vi "ImportScan.vi"(8 "error in (no error)":errorcluster, 9 "reference":refnum<vi>, 11 "Database in":refnum<class "Database.lvclass">) -> (0 "error out":errorcluster, 1 "reference 2":refnum<vi>, 3 "Database out":refnum<class "Database.lvclass">)   [LabVIEW 2014, in "Database.lvclass"]
uses:
  Database.lvclass
  Database.lvclass/Database.ctl
  <vilib>/addons/database/NI_Database_API.lvlib
panel:
  in  "scan":T1
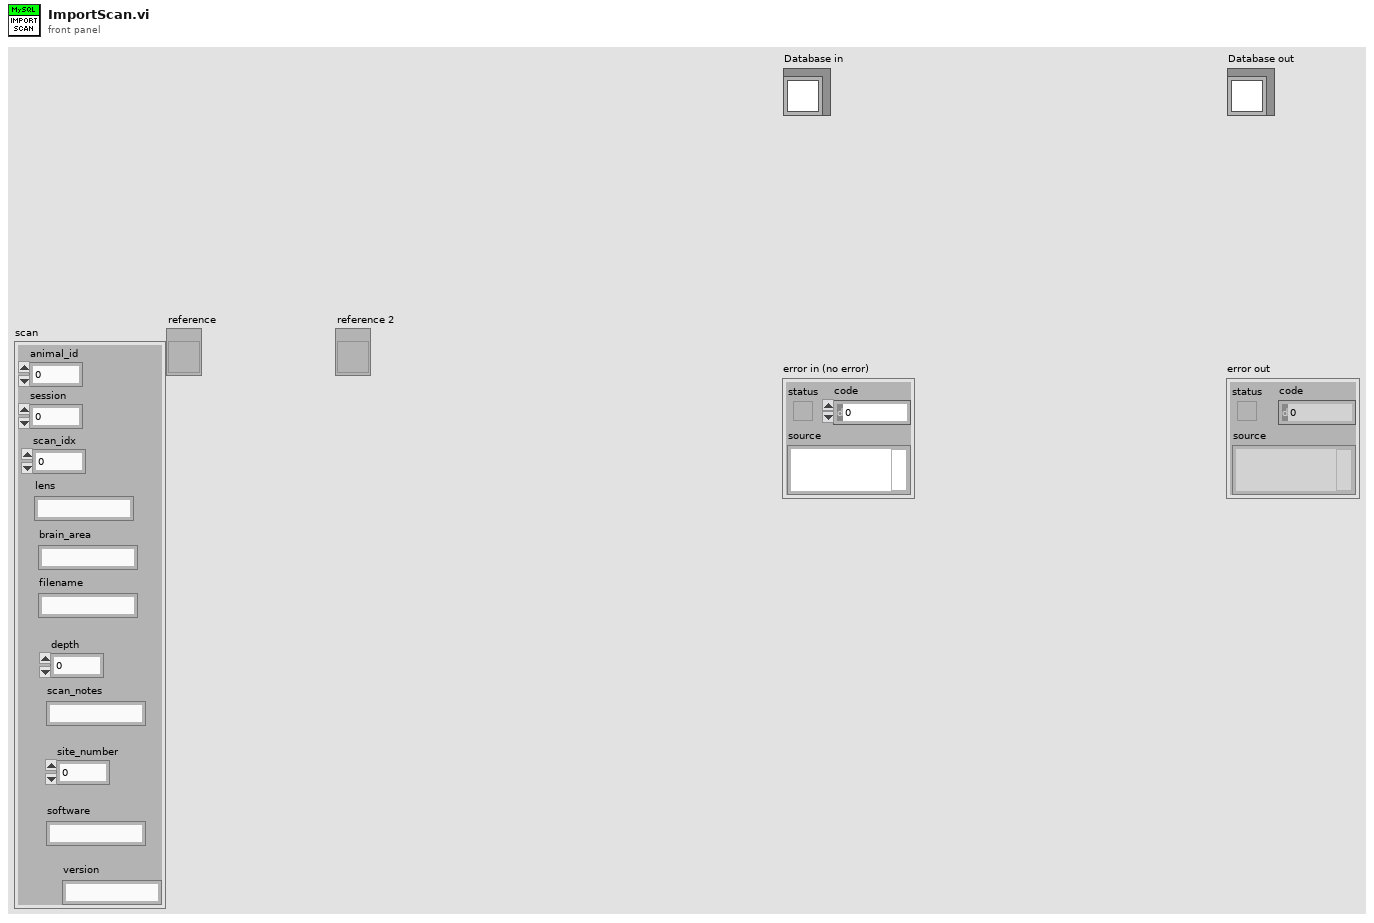
[diagram p1: front panel]
types:
  T1 = cluster{"animal_id":dbl, "session":dbl, "scan_idx":dbl, "lens":string, "brain_area":string, "filename":string, "depth":dbl, "scan_notes":string, "site_number":dbl, "software":string, "version":string}
  T2 = typedef "NI_Database_API.lvlib/Conn ObjectReference.ctl" = refnum<k1>
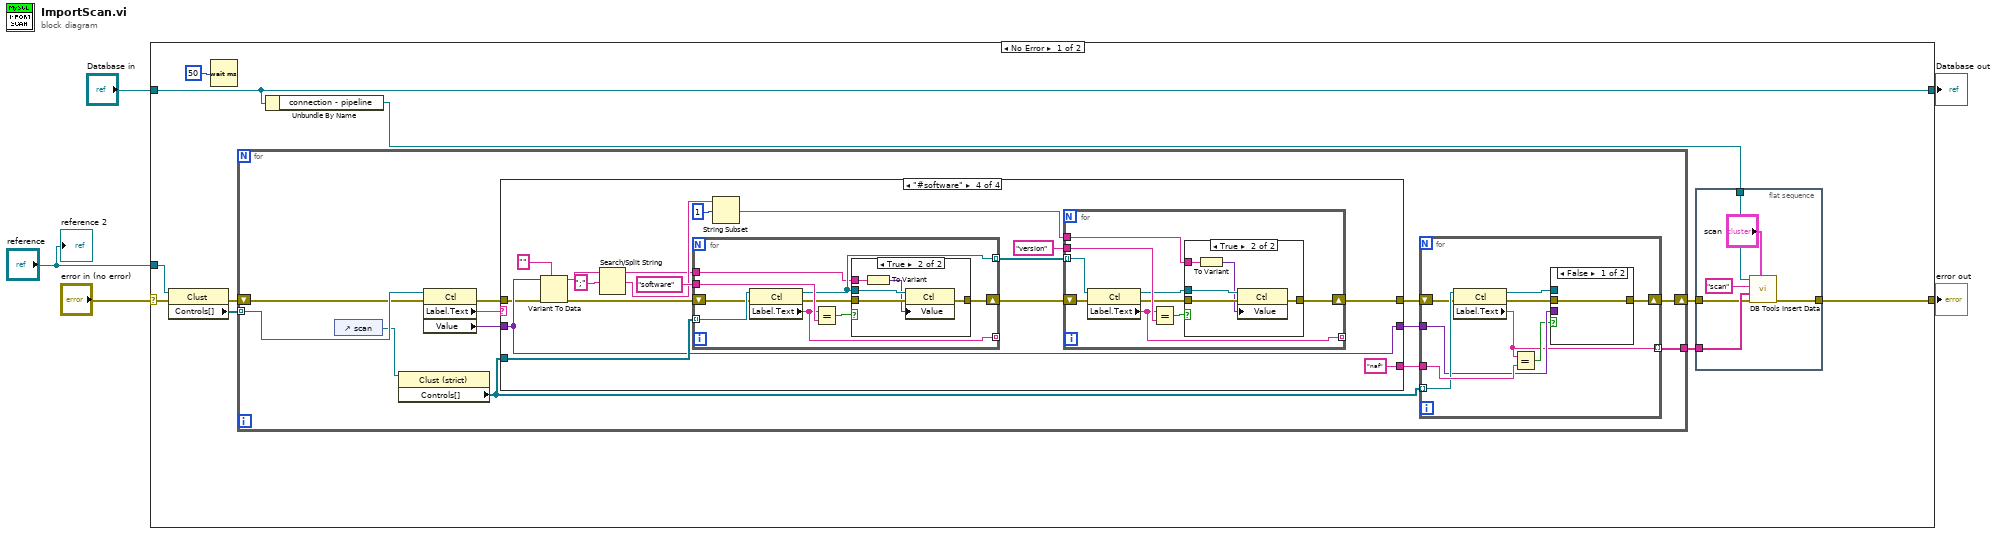
[diagram p0: block diagram]
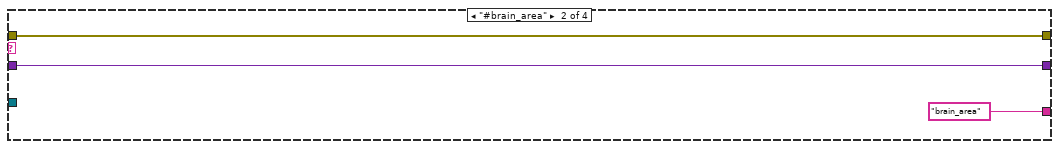
[diagram p3: hidden frame]
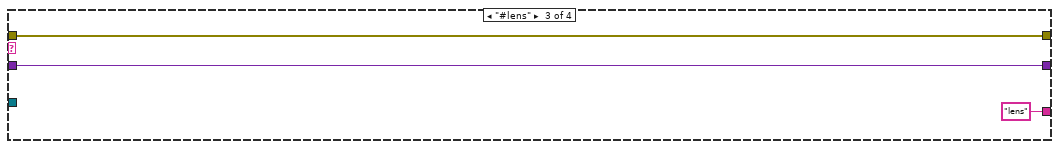
[diagram p4: hidden frame]
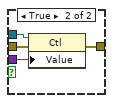
[diagram p7: hidden frame]
diagram:
  n1 = case shown="No Error" "error in (no error)" {
    selector: "error in (no error)" -> [w10 w105]
    tunnel: [w7 w105] -> w4
    tunnel: [w9 w104] -> w2
    tunnel: "Database in" -> [w9 w104]
    tunnel: "reference" -> [w6 _]
    frame No Error {
      n2 = property class="Clust"(reference=w6, error in=w10) -> (error out=w14:errorcluster, "Controls[]"=w15:refnum<vi>[])  [unwired: 1 out]
      n3 = Wait (ms)(milliseconds to wait=u32 50) -> ()  [unwired: 1 out]
      n4 = for {
        tunnel: w15 -> [w33] mode=indexing
        shift-right: [w22] -> w11
        shift-left: w14 -> [w32]
        tunnel: [w30] -> w13
        n5 = control-ref of="scan"() -> (w31:refnum<vi>)
        n6 = property class="Clust (strict)"(reference=w31) -> ("Controls[]"=w23:refnum<vi>[])  [unwired: 1 in, 2 out]
        n7 = property class="Ctl"(reference=w33, error in=w32) -> (error out=w28:errorcluster, "Label.Text"=w29:string, "Value"=w26:variant)  [unwired: 1 out]
        n8 = case shown="\"#software\"" w29 {
          selector: w29 -> [w36 _ _ _]
          tunnel: [w36 "brain_area" ("session") "lens" ("session") "naf" ("session")] -> w24
          tunnel: w28 -> [w34 w37 w40 w50]
          tunnel: [w34 w37 w40 w55] -> w27
          tunnel: w26 -> [w35 w38 w41 w52]
          tunnel: [w35 w38 w41 w52] -> w25
          tunnel: w23 -> [_ _ _ w58]
          frame "False", Default {
          }
          frame "#brain_area" {
          }
          frame "#lens" {
          }
          frame "#software" {
            n9 = Variant To Data(error in=w50, type="", Variant=w52) -> (data=w45:string, error out=w49:errorcluster)
            n10 = Search/Split String(string=w45, search string/char (-)=";") -> (substring before match=w44:string, match + rest of string=w47:string)  [unwired: 1 in, 1 out]
            n11 = for {
              tunnel: "software" ("session") -> [w83]
              tunnel: w58 -> [w82] mode=indexing
              tunnel: [w80] -> _ mode=indexing
              shift-right: [w77] -> w53
              shift-left: w49 -> [w79]
              tunnel: [w76] -> w54 mode=indexing
              tunnel: w44 -> [w75]
              n12 = property class="Ctl"(reference=w82, error in=w79) -> (reference out=w76:refnum<vi>, error out=w78:errorcluster, "Label.Text"=w80:string)
              n13 = Equal?(x=w80, y=w83) -> (x = y?=w81:bool)
              n14 = case shown="True" w81 {
                tunnel: w76 -> [_ w89]
                tunnel: w78 -> [w84 w88]
                tunnel: [w84 w87] -> w77
                tunnel: w75 -> [_ w85]
                frame False {
                }
                frame True {
                  n15 = To Variant(anything=w85) -> (Variant=w86:variant)
                  n16 = property class="Ctl"(reference=w89, error in=w88, "Value"=w86) -> (error out=w87:errorcluster)  [unwired: 1 out]
                }
              }
            }
            n17 = String Subset(string=w47, offset (0)=1) -> (substring=w43:string)  [unwired: 1 in]
            n18 = for {
              tunnel: "version" ("session") -> [w68]
              tunnel: w54 -> [w67] mode=indexing
              tunnel: [w64] -> _ mode=indexing
              shift-right: [w62] -> w55
              shift-left: w53 -> [w61]
              tunnel: w43 -> [w60]
              n19 = property class="Ctl"(reference=w67, error in=w61) -> (reference out=w66:refnum<vi>, error out=w63:errorcluster, "Label.Text"=w64:string)
              n20 = Equal?(x=w64, y=w68) -> (x = y?=w65:bool)
              n21 = case shown="True" w65 {
                tunnel: w66 -> [_ w74]
                tunnel: w63 -> [w69 w73]
                tunnel: [w69 w72] -> w62
                tunnel: w60 -> [_ w70]
                frame False {
                }
                frame True {
                  n22 = To Variant(anything=w70) -> (Variant=w71:variant)
                  n23 = property class="Ctl"(reference=w74, error in=w73, "Value"=w71) -> (error out=w72:errorcluster)  [unwired: 1 out]
                }
              }
            }
          }
        }
        n24 = for {
          tunnel: w24 -> [w98]
          tunnel: w25 -> [w95]
          tunnel: w23 -> [w97] mode=indexing
          tunnel: [w93] -> w30 mode=indexing
          shift-right: [w91] -> w22
          shift-left: w27 -> [w90]
          n25 = property class="Ctl"(reference=w97, error in=w90) -> (reference out=w96:refnum<vi>, error out=w92:errorcluster, "Label.Text"=w93:string)
          n26 = Equal?(x=w93, y=w98) -> (x = y?=w94:bool)
          n27 = case shown="False" w94 {
            tunnel: w96 -> [_ w103]
            tunnel: w95 -> [_ w102]
            tunnel: w92 -> [w99 w101]
            tunnel: [w99 w100] -> w91
            frame False {
            }
            frame True {
              n28 = property class="Ctl"(reference=w103, error in=w101, "Value"=w102) -> (error out=w100:errorcluster)  [unwired: 1 out]
            }
          }
        }
      }
      n29 = Unbundle By Name(w9) -> ("connection - pipeline"=w12:T2)
      n30 = flat-sequence {
        tunnel: w13 -> [w21]
        tunnel: w12 -> [w20]
        tunnel: w11 -> [w19]
        tunnel: [w17] -> w7
        frame #0 {
          n31 = call <vilib>:"DB Tools Insert Data.vi"("data"="scan", "error in (no error)"=w19, "columns"=w21, "table"="scan" ("session"), "connection reference"=w20) -> ("error out"=w17:errorcluster)  [unwired: 5 in, 1 out]
        }
      }
    }
    frame Error {
    }
  }
  "error out" <- w4
  "Database out" <- w2
  "reference 2" <- "reference"
